vi "Statistics calculation real-time A.vi"(10 "Reset calc":bool, 11 "new data":dbl) -> (2 "Statistics":cluster{"Count":i32, "Mean":dbl, "Std":dbl} {"Std" format="%#_6p"; "Mean" format="%#_6p"}, 3 "Histogram Graph":T1)   [LabVIEW 2019]
uses:
  <vilib>/ptbypt/NI_PtbyPt.lvlib
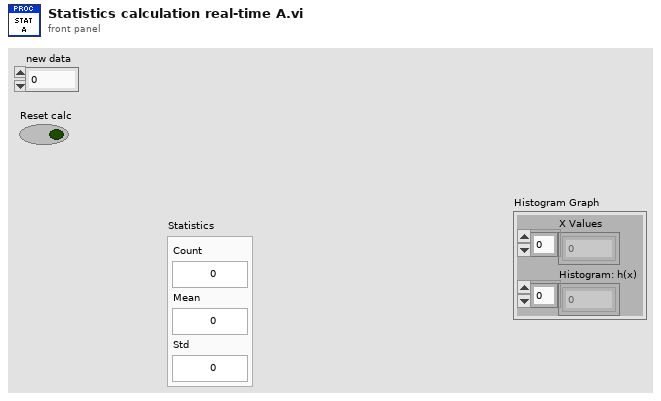
[diagram p1: front panel]
types:
  T1 = cluster{"X Values":dbl[], "Histogram: h(x)":i32[]}
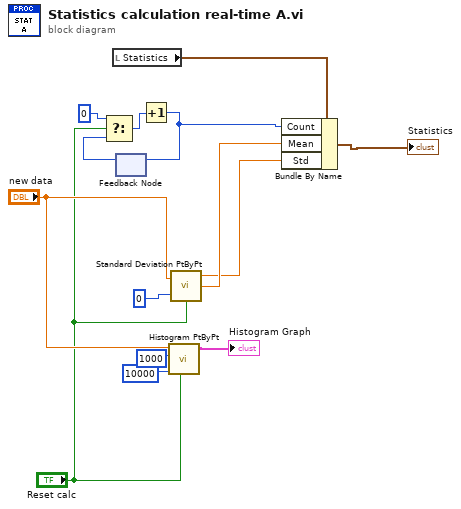
[diagram p0: block diagram]
diagram:
  n1 = local read "Statistics"() -> (w5:cluster{"Count":i32, "Mean":dbl, "Std":dbl})
  n2 = feedback #1() -> (w7:i32)  [unwired: 1 in]
  n3 = Select(t=0, s="Reset calc", f=w7) -> (s? t:f=w6:i32)
  n4 = Increment(x=w6) -> (x+1=w4:i32)
  n5 = feedback-in #1(w4) -> ()
  n6 = call <vilib>:"Histogram PtByPt.vi"("initialize"="Reset calc", "sample length"=10000, "intervals"=1000, "x"="new data") -> ("Histogram Graph"=→"Histogram Graph":T1)  [unwired: 4 in, 3 out]
  n7 = call <vilib>:"Standard Deviation PtByPt.vi"("x"="new data", "sample length"=0, "initialize"="Reset calc") -> ("standard deviation"=w2:dbl, "mean"=w3:dbl)  [unwired: 1 out]
  n8 = Bundle By Name(cluster=w5, "Count"=w4, "Mean"=w3, "Std"=w2) -> (→"Statistics":cluster{"Count":i32, "Mean":dbl, "Std":dbl})
